vi "Configure Modulation (PSK).vi"(0 "VISA resource name":refnum<visa-resource-name>, 1 "Enable PSK Modulation (T:Enable)":bool=TRUE, 5 "PSK Source (0: Internal)":u16(ring) items=["Internal", "External"], 7 "Channel (1:Channel 1)":i32(ring)=1 items=["Channel 1"=1, "Channel 2"=2], 9 "Polarity (0: Positive)":u16(ring) items=["Positive", "Negative"], 11 "error in (no error)":errorcluster, 12 "Key Frequency (100.000 Hz)":dbl=100.0 format="%.3f") -> (4 "VISA resource name out":refnum<visa-resource-name>, 15 "error out":errorcluster)   [LabVIEW 2023, in "Siglent SDG X Series.lvlib"]
doc: "Configures and enables PSK modulation for the SDG2000X/E series.\n\n<B>Note:</B> The carrier waveform shape and parameters are set by the Configure Standard Waveform VI."
uses:
  Siglent SDG X Series.lvlib
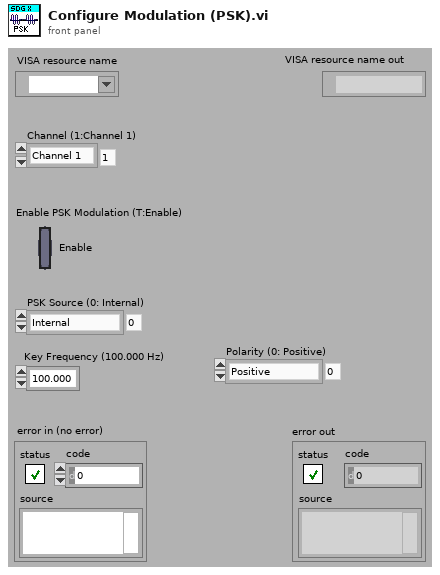
[diagram p1: front panel]
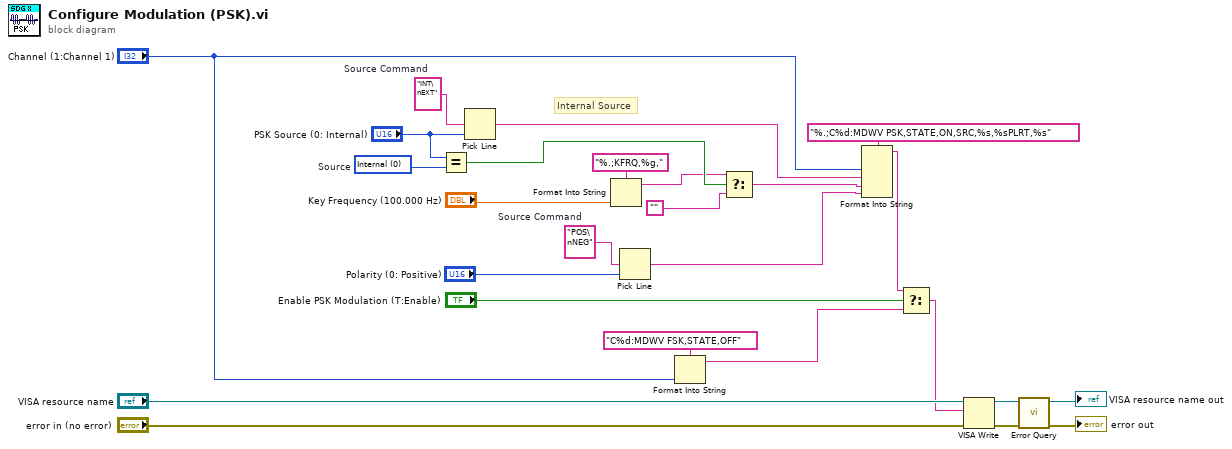
[diagram p0: block diagram]
diagram:
  w7 = "POS\nNEG"  # Source Command
  w19 = "INT\nEXT"  # Source Command
  w17 = u16 0 items=["Internal", "External"]  # Source
  # "Internal Source"
  n1 = Equal?(x="PSK Source (0: Internal)", y=w17) -> (x = y?=w3:bool)
  n2 = Pick Line(multi-line string=w19, line index="PSK Source (0: Internal)") -> (output string=w15:string)  [unwired: 1 in]
  n3 = Format Into String(format string="%.;KFRQ,%g,", "Key Frequency (100.000 Hz)") -> (resulting string=w2:string)  [unwired: 2 in, 1 out]
  n4 = Pick Line(multi-line string=w7, line index="Polarity (0: Positive)") -> (output string=w6:string)  [unwired: 1 in]
  n5 = Format Into String(format string="C%d:MDWV FSK,STATE,OFF", "Channel (1:Channel 1)") -> (resulting string=w12:string)  [unwired: 2 in, 1 out]
  n6 = Select(t=w2, s=w3, f="") -> (s? t:f=w4:string)
  n7 = Format Into String(format string="%.;C%d:MDWV PSK,STATE,ON,SRC,%s,%sPLRT,%s", "Channel (1:Channel 1)", w15, w4, w6) -> (resulting string=w11:string)  [unwired: 2 in, 1 out]
  n8 = Select(t=w11, s="Enable PSK Modulation (T:Enable)", f=w12) -> (s? t:f=w10:string)
  n9 = VISA Write(VISA resource name="VISA resource name", write buffer=w10, error in (no error)="error in (no error)") -> (VISA resource name out=w24:refnum<visa-resource-name>, error out=w23:errorcluster)  [unwired: 1 out]
  n10 = call "Error Query.vi"("error in (no error)"=w23, "VISA resource name"=w24) -> ("error out"=→"error out":errorcluster, "VISA resource name out"=→"VISA resource name out":refnum<visa-resource-name>)  [unwired: 6 in, 2 out]
